vi "GlobalGetPhysikalInstrumentsOnOff.vi"() -> ()   [LabVIEW 2011]
panel:
  out "GetMirror":bool
  out "GetScanner":bool
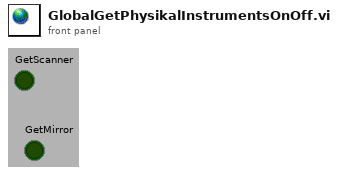
[diagram p1: front panel]
diagram:
